vi "cccc.vi"(1 "error in 2":errorcluster) -> (0 "error out 2":errorcluster)   [LabVIEW 2016]
panel:
  out "Final Result":string[][](array[string])
  out "Cycle data by seq":dbl[][][](array[numeric])
  out "sequence result header 2":string[](array[string])
  out "Final result header":string[](array[string])
  out "sequence result header":string[](array[string])
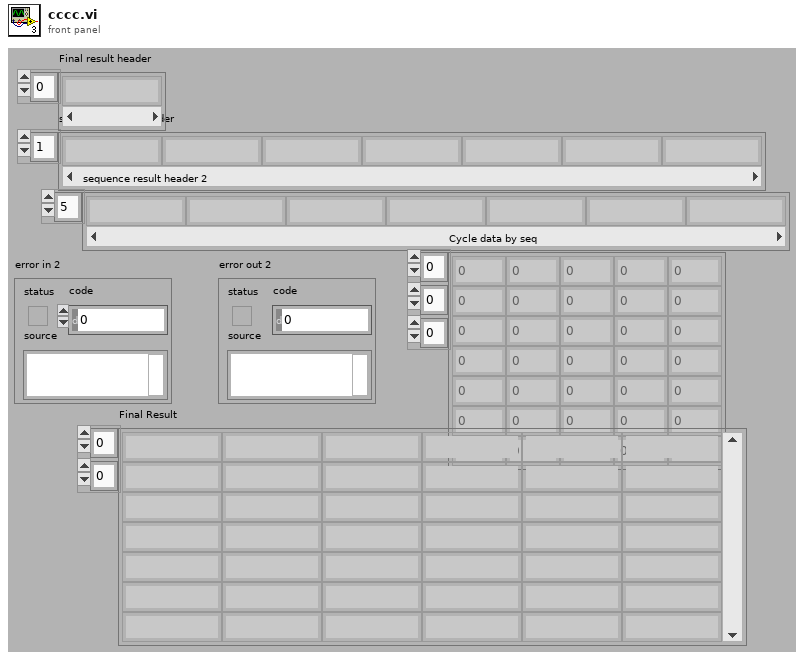
[diagram p1: front panel]
types:
  T1 = typedef "data control cluster.ctl" = cluster{"Final result header":string[], "sequence result header":string[], "cycle result header ":string[], "Final Result":string[][], "sequence  Result":dbl[][], "Cycle data by seq":dbl[][][], "Cycle data by position":dbl[][][], "Final seq  Result":dbl[][], "only specific type":dbl[][]}
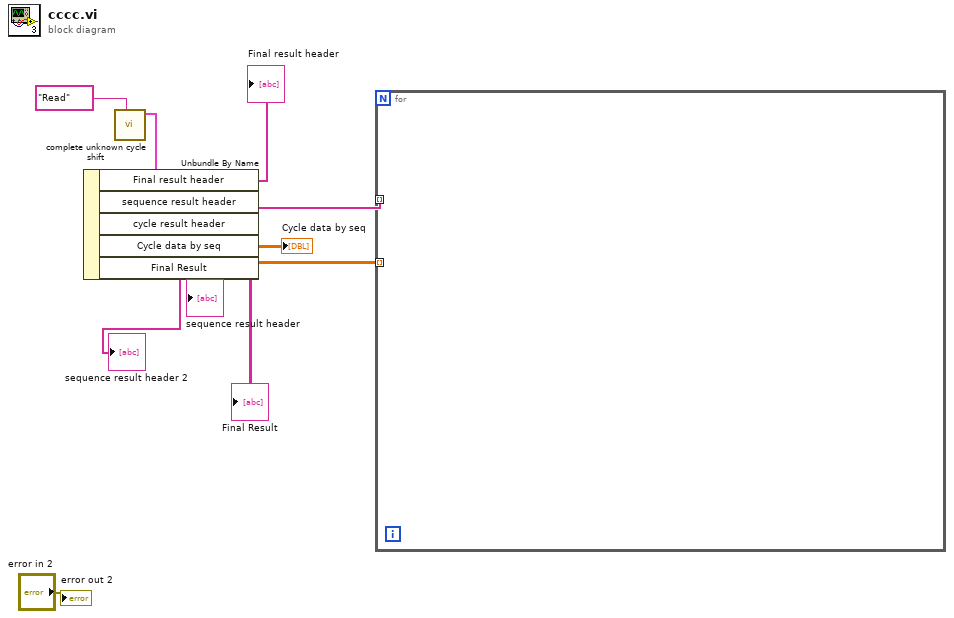
[diagram p0: block diagram]
diagram:
  n1 = call "complete unknown cycle shift.vi"("read write shift"="Read") -> ("DATA CLUSTER out"=w6:T1)  [unwired: 9 in, 1 out]
  n2 = Unbundle By Name(w6) -> ("Final result header"=→"Final result header":string[], "sequence result header"=w5:string[], "cycle result header"=→"sequence result header 2":string[], "Cycle data by seq"=w2:dbl[][][], "Final Result"=→"Final Result":string[][])
  "sequence result header" <- w5
  "Cycle data by seq" <- w2
  n3 = for {
    tunnel: w5 -> [_] mode=indexing
    tunnel: w2 -> [_] mode=indexing
  }
  "error out 2" <- "error in 2"
